vi "Enumerate Processes.vi"(4 "error in (no error)":errorcluster) -> (0 "error out":errorcluster, 2 "Process Count":i32, 3 "Process IDs":i32[](array[numeric]))   [LabVIEW 2011]
uses:
  psapi.dll
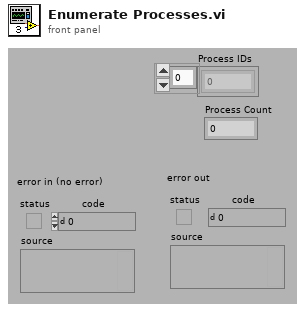
[diagram p1: front panel]
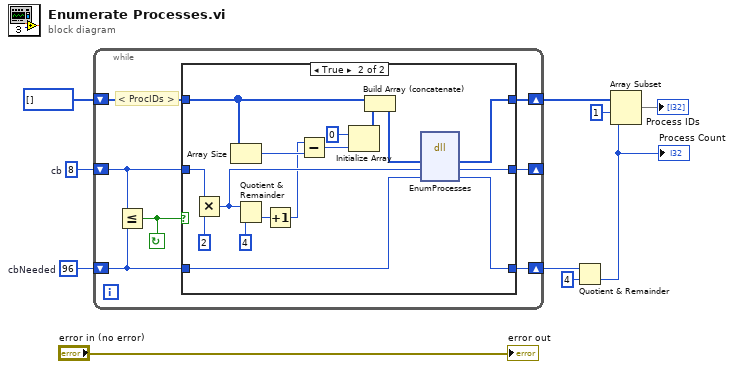
[diagram p0: block diagram]
diagram:
  w10 = 8  # cb
  w9 = 96  # cbNeeded
  n1 = while {
    shift-right: [w15] -> _
    shift-left: w10 -> [w16]
    shift-right: [w13] -> w7
    shift-left: w9 -> [w14]
    shift-right: [w11] -> w5
    shift-left: i32[] [] ("initialized array") -> [w12]
    stop <- w17 continue-if-true
    # "< ProcIDs >"
    n2 = Less Or Equal?(x=w16, y=w14) -> (x <= y?=w17:bool)
    n3 = case shown="True" w17 {
      tunnel: w16 -> [w20 w36]
      tunnel: [w20 w30] -> w15
      tunnel: w14 -> [w19 w33]
      tunnel: [w19 w32] -> w13
      tunnel: w12 -> [w18 w28]
      tunnel: [w18 w26] -> w11
      frame False {
      }
      frame True {
        n4 = Multiply(x=w36, y=2) -> (x*y=w31:i32)
        n5 = Array Size(array=w28) -> (size(s)=w24:i32)
        n6 = Quotient & Remainder(x=w31, y=4) -> (floor(x/y)=w22:i32)  [unwired: 1 out]
        n7 = Increment(x=w22) -> (x+1=w21:i32)
        n8 = Subtract(x=w21, y=w24) -> (x-y=w23:i32)
        n9 = Initialize Array(0 ("cbNeeded"), w23) -> (w25:i32[])
        n10 = Build Array (concatenate)(w28, w25) -> (w27:i32[])
        n11 = dll-call lib="psapi.dll" fn="EnumProcesses"("lpidProcess"=w27, "cb"=w31, "cbNeeded"=w33) -> ("lpidProcess"=w26:i32[], "cb"=w30:i32, "cbNeeded"=w32:i32)  [unwired: 3 in, 3 out]
      }
    }
  }
  n12 = Quotient & Remainder(x=w7, y=4) -> (floor(x/y)=w3:i32)  [unwired: 1 out]
  "Process Count" <- w3
  n13 = Array Subset(array=w5, index=1, length=w3) -> (→"Process IDs":i32[])
  "error out" <- "error in (no error)"
